vi "self-balance_interface.vi"() -> ()   [LabVIEW 2019]
uses:
  65a3cf9d-86d2-4813-94bd-8b89f2547100.vi
  1c29e484-c04a-4e29-ad32-b5bb79577eec.vi
  <vilib>/Instr/_visa.llb/VISA Configure Serial Port (Instr).vi
  <vilib>/express/express shared/transition.llb/Dynamic To Waveform Array.vi
  <vilib>/express/express signal manip/GetorSetDDTAttributes/Set DDT Attributes/SetT0.vi
  <vilib>/express/express shared/transition.llb/Waveform Array To Dynamic.vi
  <vilib>/express/express signal manip/GetorSetDDTAttributes/Set DDT Attributes/Set DDT Properties.xnode
panel:
  in  "baud rate (9600)":u32=115200
  in  "Salva su Excel":bool
  in  "Percorso file":path=path "C:/Users/d.bevilacqua/Desktop/Bil.xlsx"
  in  "contatore_loop":i32=100
  in  "Tab Control":T1(tab)
  out "Accellerometro":dbl(knob) scale=-90.0..90.0
  out "Filtro complementare:":dbl caption="gradi"
  out "Accellerometro:":dbl caption="gradi"
  out "Correzione baricentro:":sgl caption="gradi" format="%#.1f"
  out "Baricentro":dbl(knob) scale=-15.0..15.0
  out "Controllo:":bool
  out "Angolo":dbl(knob)=-0.787992585102927 scale=-30.0..30.0
  out "Batteria":dbl(slide) scale=11.2..12.6
  out "Velocità motori":dbl(knob) scale=-100.0..100.0
  out "Velocità angolare:":dbl(slide) scale=-300.0..300.0
  out "Motori:":dbl caption="%"
  out "Batteria:":dbl caption="Volts" format="%#_3g"
  out "Giroscopio:":dbl caption="gradi/s"
  in  "Frequenza campionamento dati":i32=120 caption="ms" min=48 max=2400 step=1
  out "Traccia batteria":ext(graph)
  out "Traccia errore":ext(graph)
  out "Traccia angolo":cluster{dbl, dbl, dbl}(graph)
  out "Traccia varianza":ext(graph)
  out "Traccia media":cluster{ext, ext}(graph)
  out "Media errore:":dbl format="%.1e"
  out "Varianza errore:":dbl format="%#_2e"
  out "Errore istantaneo:":dbl format="%#_2g"
  in  "Indietro":bool
  in  "Stop":bool
  in  "Destra":bool
  in  "Sinistra":bool
  in  "Avanti":bool
  in  "Proporzionale":sgl(slide)=20.0 min=0 max=35 step=0.1 scale=0.0..35.0 scale format="%#_3f"
  in  "Integrativo":sgl(slide)=1.4699999 min=0 max=2 step=0.01 scale=0.0..2.0 scale format="%#_2f"
  in  "Derivativo":dbl(slide)=50.31000000000001 min=0.0 max=70.0 step=0.01 scale=0.0..70.0 scale format="%#_2f"
  in  "Applica":bool
  in  "Accensione motori":bool=TRUE caption="motori"
  in  "Applica 3":bool
  in  "Applica 2":bool
  out "Lettura Seriale":string
  in  "stop":bool
  in  "PORTA SERIALE":refnum<visa-resource-name>
  # "BIL 6.0"
  # "Inclinazione"
  # "Media e Varianza dell'errore"
  # "Configurazione PID"
  # "Pilotaggio manuale"
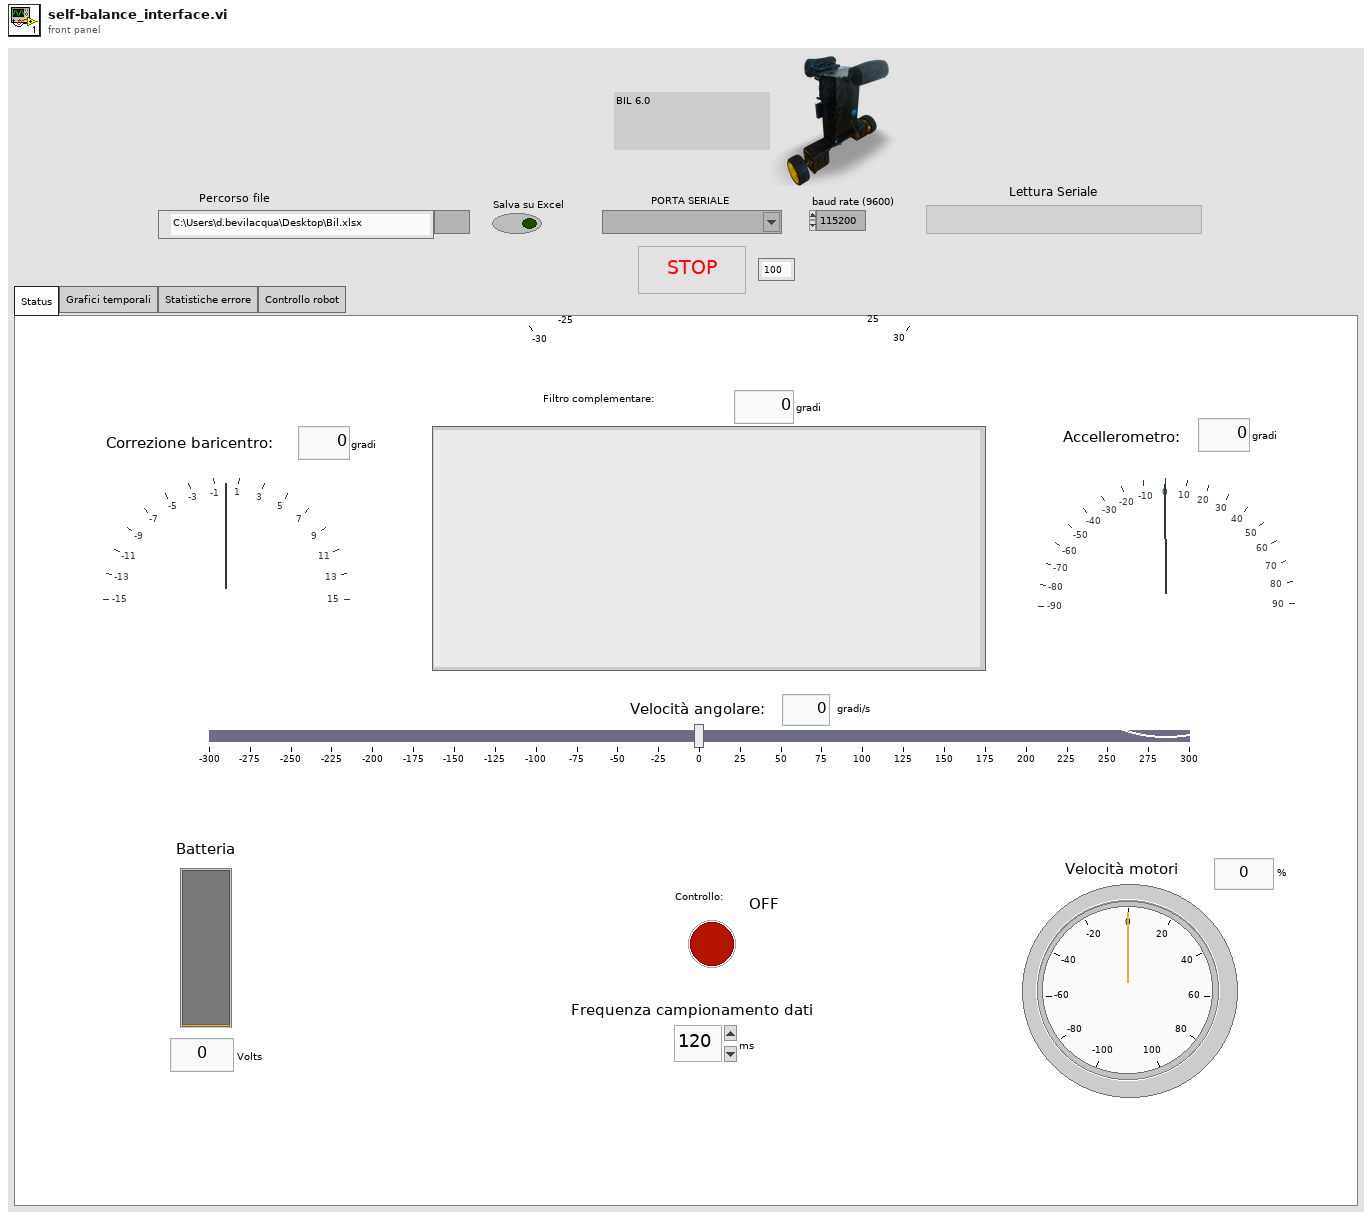
[diagram p1: front panel]
types:
  T1 = enum32{"Status", "Grafici temporali", "Statistiche errore", "Controllo robot"}
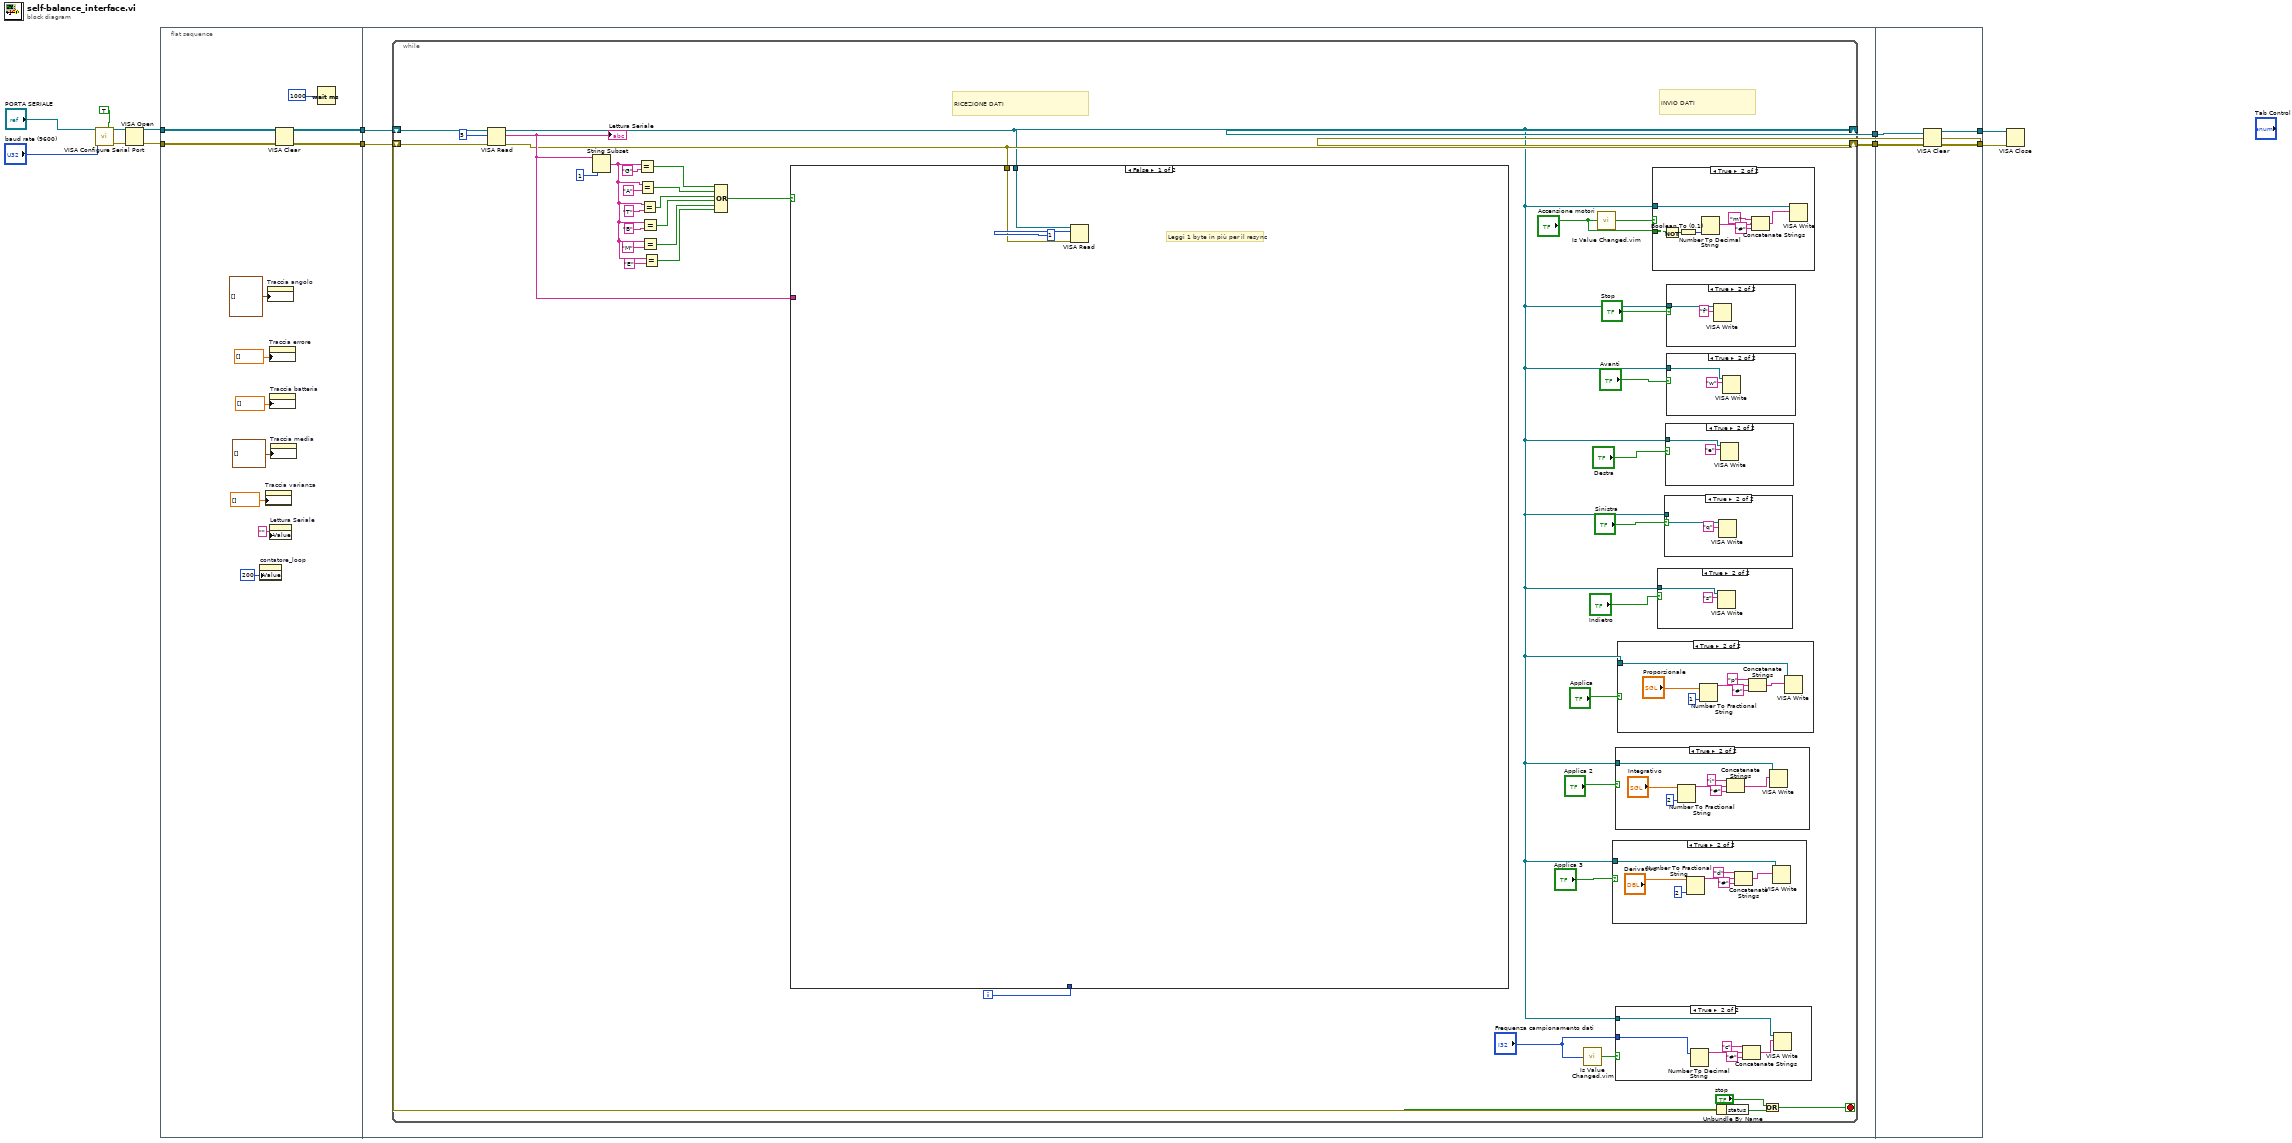
[diagram p0: block diagram]
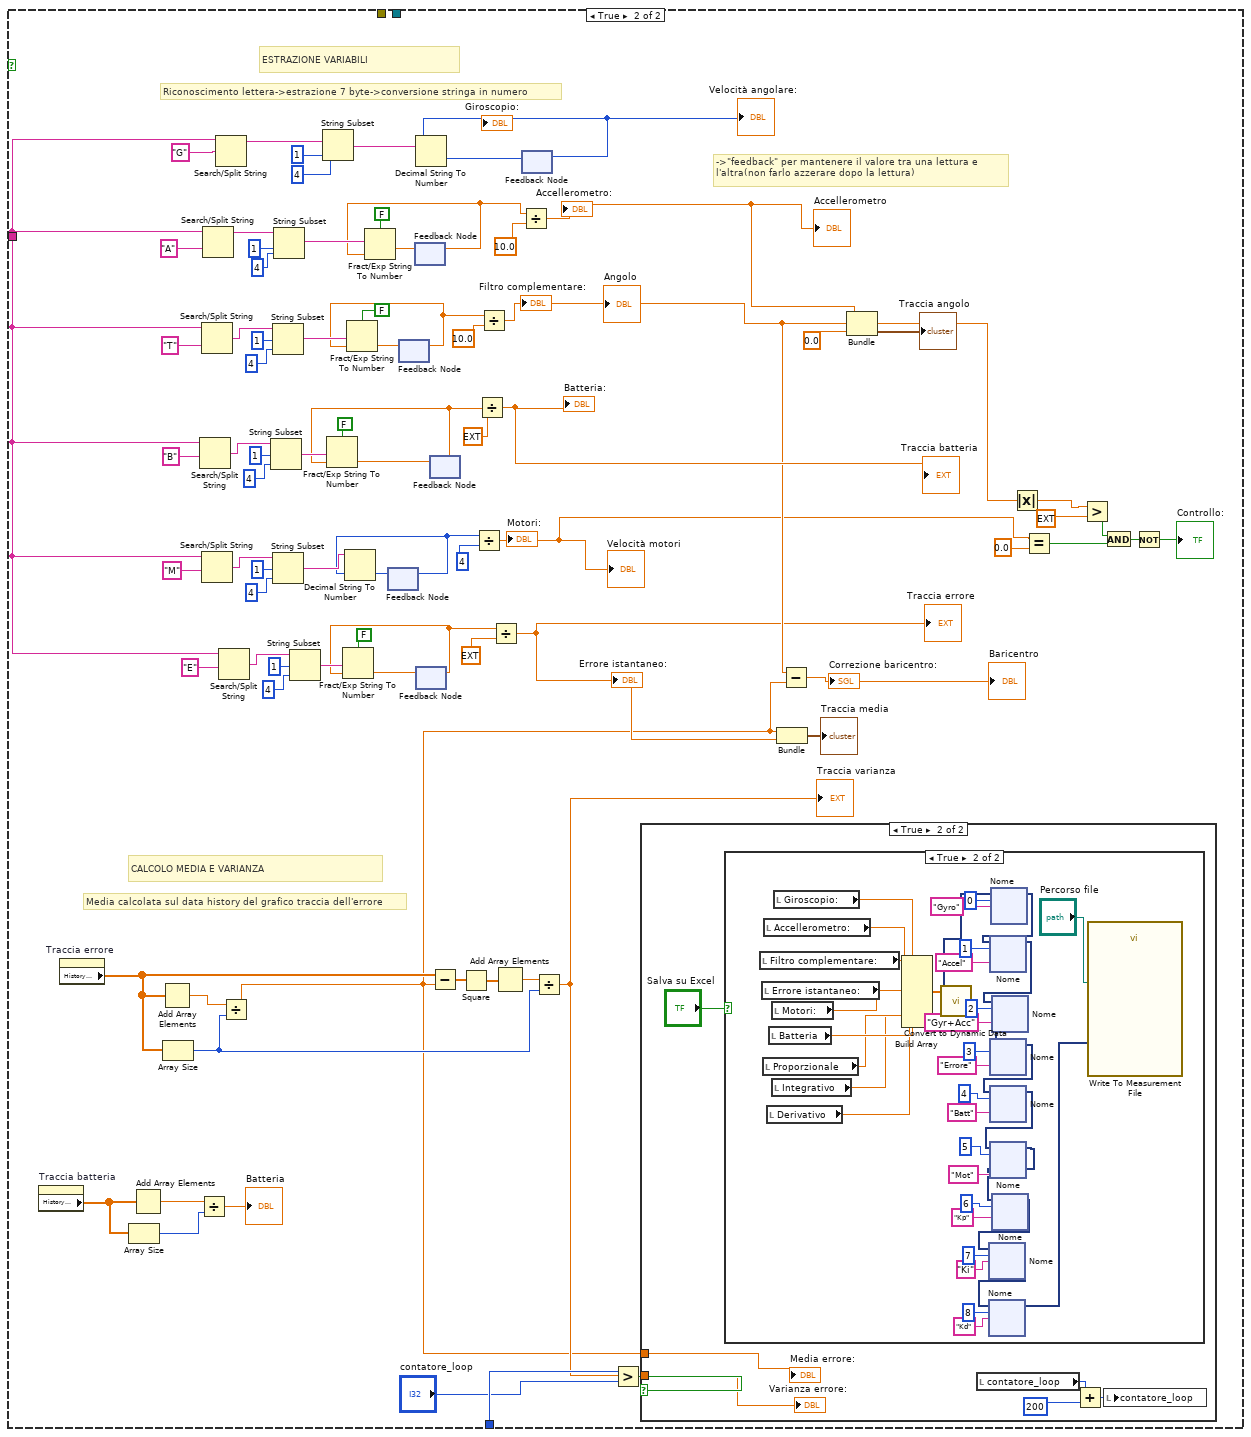
[diagram p10: hidden frame]
diagram:
  n1 = call-poly "VISA Configure Serial Port"("VISA resource name"="PORTA SERIALE", "Enable Termination\nChar (T)"=TRUE, "baud rate (9600)"="baud rate (9600)") -> ("VISA resource name out"=w12:refnum<visa-resource-name>, "error out"=w11:errorcluster)  [unwired: 11 in]
  n2 = VISA Open(error in (no error)=w11, VISA resource name=w12) -> (VISA resource name=w9:refnum<visa-resource-name>, error out=w8:errorcluster)  [unwired: 3 in]
  n3 = flat-sequence {
    tunnel: [w16] -> w3
    tunnel: w9 -> [w24]
    tunnel: w8 -> [w23]
    tunnel: [w15] -> w2
    tunnel: [w27] -> w5
    tunnel: [w26] -> w4
    tunnel: w3 -> [w29]
    tunnel: w2 -> [w28]
    tunnel: [w360] -> w6
    tunnel: [w363] -> w7
    tunnel: w5 -> [w362]
    tunnel: w4 -> [w361]
    frame #0 {
      n4 = property on="contatore_loop" class="DigNum (strict)"("Value"=200 ("contatore_loop")) -> ()  [unwired: 2 in, 2 out]
      n5 = property on="Traccia varianza" class="WFChart (strict)"("History Data"=ext[] []) -> ()  [unwired: 2 in, 2 out]
      n6 = property on="Traccia angolo" class="WFChart (strict)"("History Data"=cluster{ext, ext, dbl}[] []) -> ()  [unwired: 2 in, 2 out]
      n7 = property on="Traccia errore" class="WFChart (strict)"("History Data"=ext[] []) -> ()  [unwired: 2 in, 2 out]
      n8 = property on="Traccia batteria" class="WFChart (strict)"("History Data"=ext[] []) -> ()  [unwired: 2 in, 2 out]
      n9 = property on="Lettura Seriale" class="Str"("Value"="" ("Lettura Seriale")) -> ()  [unwired: 2 in, 2 out]
      n10 = property on="Traccia media" class="WFChart (strict)"("History Data"=cluster{ext, ext}[] []) -> ()  [unwired: 2 in, 2 out]
      n11 = VISA Clear(VISA resource name=w24, error in (no error)=w23) -> (VISA resource name out=w16:refnum<visa-resource-name>, error out=w15:errorcluster)
      n12 = Wait (ms)(milliseconds to wait=u32 1000) -> ()  [unwired: 1 out]
    }
    frame #1 {
      n13 = while {
        shift-right: [w30] -> w27
        shift-left: w29 -> [w65]
        shift-right: [w45] -> w26
        shift-left: w28 -> [w64]
        i -> [w44]
        stop <- w41 stop-if-true
        # "RICEZIONE DATI"
        # "INVIO DATI"
        n14 = VISA Read(VISA resource name=w65, byte count=u32 5, error in (no error)=w64) -> (VISA resource name out=w30:refnum<visa-resource-name>, read buffer=w60:string, error out=w45:errorcluster)  [unwired: 1 out]
        "Lettura Seriale" <- w60
        n15 = String Subset(string=w60, length (rest)=1 ("length (rest)")) -> (substring=w52:string)  [unwired: 1 in]
        n16 = Equal?(x=w52, y="G") -> (x = y?=w58:bool)
        n17 = Equal?(x=w52, y="A") -> (x = y?=w51:bool)
        n18 = Equal?(x=w52, y="T") -> (x = y?=w50:bool)
        n19 = Equal?(x=w52, y="B") -> (x = y?=w49:bool)
        n20 = Equal?(x=w52, y="M") -> (x = y?=w48:bool)
        n21 = Equal?(x=w52, y="E") -> (x = y?=w47:bool)
        n22 = Compound Arithmetic op=OR(w58, w51, w50, w49, w48, w47) -> (w46:bool)
        n23 = case shown="False" w46 {
          tunnel: w60 -> [_ w136]
          tunnel: w30 -> [w98 _]
          tunnel: w45 -> [w97 _]
          tunnel: w44 -> [_ w112]
          frame False {
            # "Leggi 1 byte in più per il resync"
            n24 = VISA Read(VISA resource name=w98, byte count=u32 1, error in (no error)=w97) -> ()  [unwired: 4 out]
          }
          frame True {
            # "->\"feedback\" per mantenere il valore tra una lettura e l'altra(non farlo azzerare dopo la lettura)"
            # "Media calcolata sul data history del grafico traccia dell'errore"
            # "CALCOLO MEDIA E VARIANZA"
            # "Riconoscimento lettera->estrazione 7 byte->conversione stringa in numero"
            # "ESTRAZIONE VARIABILI"
            n25 = property on="Traccia batteria" class="WFChart (strict)"() -> ("History Data"=w118:ext[])  [unwired: 2 in, 2 out]
            n26 = property on="Traccia errore" class="WFChart (strict)"() -> ("History Data"=w113:ext[])  [unwired: 2 in, 2 out]
            n27 = Array Size(array=w118) -> (size(s)=w119:i32)
            n28 = Add Array Elements(numeric array=w118) -> (sum=w120:ext)
            n29 = Add Array Elements(numeric array=w113) -> (sum=w168:ext)
            n30 = Array Size(array=w113) -> (size(s)=w166:i32)
            n31 = Divide(x=w120, y=w119) -> (x/y=→"Batteria":ext)
            n32 = Search/Split String(string=w136, search string/char (-)="B") -> (match + rest of string=w173:string)  [unwired: 1 in, 2 out]
            n33 = Search/Split String(string=w136, search string/char (-)="T") -> (match + rest of string=w177:string)  [unwired: 1 in, 2 out]
            n34 = Search/Split String(string=w136, search string/char (-)="M") -> (match + rest of string=w162:string)  [unwired: 1 in, 2 out]
            n35 = Search/Split String(string=w136, search string/char (-)="A") -> (match + rest of string=w181:string)  [unwired: 1 in, 2 out]
            n36 = Search/Split String(string=w136, search string/char (-)="G") -> (match + rest of string=w155:string)  [unwired: 1 in, 2 out]
            n37 = Search/Split String(string=w136, search string/char (-)="E") -> (match + rest of string=w141:string)  [unwired: 1 in, 2 out]
            n38 = Divide(x=w168, y=w166) -> (x/y=w108:ext)
            n39 = String Subset(string=w173, offset (0)=1, length (rest)=4 ("length (rest)")) -> (substring=w148:string)
            n40 = String Subset(string=w177, offset (0)=1, length (rest)=4 ("length (rest)")) -> (substring=w149:string)
            n41 = String Subset(string=w162, offset (0)=1, length (rest)=4 ("length (rest)")) -> (substring=w159:string)
            n42 = String Subset(string=w181, offset (0)=1, length (rest)=4 ("length (rest)")) -> (substring=w158:string)
            n43 = String Subset(string=w141, offset (0)=1, length (rest)=4 ("length (rest)")) -> (substring=w137:string)
            n44 = String Subset(string=w155, offset (0)=1, length (rest)=4 ("length (rest)")) -> (substring=w156:string)
            n45 = feedback #1() -> (w145:i32)  [unwired: 1 in]
            n46 = Decimal String To Number(string=w159, default (0L)=w145) -> (number=w146:i32)  [unwired: 1 in, 1 out]
            n47 = feedback-in #1(w146) -> ()
            n48 = feedback #2() -> (w129:dbl)  [unwired: 1 in]
            n49 = Fract/Exp String To Number(use system decimal point (T)=FALSE, string=w149, default (0 dbl)=w129) -> (number=w130:dbl)  [unwired: 1 in, 1 out]
            n50 = feedback-in #2(w130) -> ()
            n51 = feedback #3() -> (w131:dbl)  [unwired: 1 in]
            n52 = Fract/Exp String To Number(use system decimal point (T)=FALSE, string=w158, default (0 dbl)=w131) -> (number=w132:dbl)  [unwired: 1 in, 1 out]
            n53 = feedback-in #3(w132) -> ()
            n54 = feedback #4() -> (w128:ext)  [unwired: 1 in]
            n55 = Fract/Exp String To Number(use system decimal point (T)=FALSE, string=w137, default (0 dbl)=w128) -> (number=w123:ext)  [unwired: 1 in, 1 out]
            n56 = feedback-in #4(w123) -> ()
            n57 = feedback #5() -> (w125:ext)  [unwired: 1 in]
            n58 = Fract/Exp String To Number(use system decimal point (T)=FALSE, string=w148, default (0 dbl)=w125) -> (number=w122:ext)  [unwired: 1 in, 1 out]
            n59 = feedback-in #5(w122) -> ()
            n60 = Subtract(x=w113, y=w108) -> (x-y=w167:ext[])
            n61 = Square(x=w167) -> (x^2=w165:ext[])
            n62 = Divide(x=w145, y=4) -> (x/y=w106:dbl)
            "Motori:" <- w106
            "Velocità motori" <- w106
            n63 = Divide(x=w125, y=ext 10.0) -> (x/y=→"Batteria:" →"Traccia batteria":ext)
            n64 = Divide(x=w129, y=10.0) -> (x/y=w116:dbl)
            "Angolo" <- w116
            "Filtro complementare:" <- w116
            n65 = Divide(x=w128, y=ext 10.0) -> (x/y=w114:ext)
            "Traccia errore" <- w114
            "Errore istantaneo:" <- w114
            n66 = Add Array Elements(numeric array=w165) -> (sum=w164:ext)
            n67 = Divide(x=w131, y=10.0) -> (x/y=w117:dbl)
            "Accellerometro" <- w117
            "Accellerometro:" <- w117
            n68 = feedback #6() -> (w143:i32)  [unwired: 1 in]
            "Giroscopio:" <- w143
            "Velocità angolare:" <- w143
            n69 = Decimal String To Number(string=w156, default (0L)=w143) -> (number=w144:i32)  [unwired: 1 in, 1 out]
            n70 = feedback-in #6(w144) -> ()
            n71 = Divide(x=w164, y=w166) -> (x/y=w109:ext)
            "Traccia varianza" <- w109
            n72 = Greater?(x=w112, y="contatore_loop") -> (0:w110:bool)
            n73 = case shown="True" w110 {
              tunnel: w108 -> [_ w185]
              tunnel: w109 -> [_ w184]
              frame False {
              }
              frame True {
                n74 = case shown="True" "Salva su Excel" {
                  frame False {
                  }
                  frame True {
                    n75 = local read "Filtro complementare:"() -> (w225:dbl)
                    n76 = local read "Errore istantaneo:"() -> (w224:dbl)
                    n77 = local read "Proporzionale"() -> (w221:sgl)
                    n78 = local read "Accellerometro:"() -> (w226:dbl)
                    n79 = local read "Derivativo"() -> (w219:dbl)
                    n80 = local read "Batteria"() -> (w222:dbl)
                    n81 = local read "Motori:"() -> (w223:dbl)
                    n82 = local read "Integrativo"() -> (w220:sgl)
                    n83 = local read "Giroscopio:"() -> (w227:dbl)
                    n84 = Build Array(w227, w226, w225, w224, w223, w222, w221, w220, w219) -> (w218:dbl[])
                    n85 = call "Convert to Dynamic Data"("Array"=w218) -> ("Dynamic Data Type"=w217:dynamicdata)  [unwired: 3 in]
                    n86 = xnode "Nome"("Signals In"=w217, "Signal Index"=0, "Signal Name"="Gyro") -> ("Signals Out"=w206:dynamicdata)  [unwired: 1 in, 1 out]
                    n87 = xnode "Nome"("Signals In"=w206, "Signal Index"=1, "Signal Name"="Accel") -> ("Signals Out"=w205:dynamicdata)  [unwired: 1 in, 1 out]
                    n88 = xnode "Nome"("Signals In"=w205, "Signal Index"=2, "Signal Name"="Gyr+Acc") -> ("Signals Out"=w204:dynamicdata)  [unwired: 1 in, 1 out]
                    n89 = xnode "Nome"("Signals In"=w204, "Signal Index"=3, "Signal Name"="Errore") -> ("Signals Out"=w203:dynamicdata)  [unwired: 1 in, 1 out]
                    n90 = xnode "Nome"("Signals In"=w203, "Signal Index"=4, "Signal Name"="Batt") -> ("Signals Out"=w199:dynamicdata)  [unwired: 1 in, 1 out]
                    n91 = xnode "Nome"("Signals In"=w199, "Signal Index"=5, "Signal Name"="Mot") -> ("Signals Out"=w197:dynamicdata)  [unwired: 1 in, 1 out]
                    n92 = xnode "Nome"("Signals In"=w197, "Signal Index"=6, "Signal Name"="Kp") -> ("Signals Out"=w194:dynamicdata)  [unwired: 1 in, 1 out]
                    n93 = xnode "Nome"("Signals In"=w194, "Signal Index"=7, "Signal Name"="Ki") -> ("Signals Out"=w193:dynamicdata)  [unwired: 1 in, 1 out]
                    n94 = xnode "Nome"("Signals In"=w193, "Signal Index"=8, "Signal Name"="Kd") -> ("Signals Out"=w192:dynamicdata)  [unwired: 1 in, 1 out]
                    n95 = call "Write To Measurement File"("Signals"=w192, "Filename"="Percorso file") -> ()  [unwired: 15 in, 3 out]
                  }
                }
                n96 = local read "contatore_loop"() -> (w187:i32)
                n97 = Add(x=w187, y=200) -> (x+y=w188:i32)
                n98 = local write "contatore_loop"(w188) -> ()
                "Media errore:" <- w185
                "Varianza errore:" <- w184
              }
            }
            n99 = Bundle(w108, w114) -> (→"Traccia media":cluster{ext, ext})  [unwired: 1 in]
            n100 = Subtract(x=w116, y=w108) -> (x-y=→"Baricentro" →"Correzione baricentro:":ext)
            n101 = Bundle(w117, w116, 0.0) -> (→"Traccia angolo":cluster{dbl, dbl, dbl})  [unwired: 1 in]
            n102 = Absolute Value(x=w116) -> (abs(x)=w104:dbl)
            n103 = Equal?(x=w106, y=0.0) -> (x = y?=w107:bool)
            n104 = Greater?(x=w104, y=ext 35.0) -> (0:w102:bool)
            n105 = And(x=w102, y=w107) -> (x .and. y?=w101:bool)
            n106 = Not(x=w101) -> (.not. x?=→"Controllo:":bool)
          }
        }
        n107 = call "Is Value Changed.vim"("value"="Frequenza campionamento dati") -> ("changed or first call?"=w32:bool)
        n108 = call "Is Value Changed.vim"("value"="Accensione motori") -> ("changed or first call?"=w63:bool)
        n109 = case shown="True" "Applica 3" {
          tunnel: w30 -> [_ w74]
          frame False {
          }
          frame True {
            n110 = Number To Fractional String(number="Derivativo", precision (6)=i16 2) -> (F-format string=w78:string)  [unwired: 2 in]
            n111 = Concatenate Strings("d" ("write buffer"), w78, "#" ("string")) -> (w73:string)
            n112 = VISA Write(VISA resource name=w74, write buffer=w73) -> ()  [unwired: 1 in, 3 out]
          }
        }
        n113 = case shown="True" "Applica 2" {
          tunnel: w30 -> [_ w81]
          frame False {
          }
          frame True {
            n114 = Number To Fractional String(number="Integrativo", precision (6)=i16 2) -> (F-format string=w85:string)  [unwired: 2 in]
            n115 = Concatenate Strings("i" ("write buffer"), w85, "#" ("string")) -> (w80:string)
            n116 = VISA Write(VISA resource name=w81, write buffer=w80) -> ()  [unwired: 1 in, 3 out]
          }
        }
        n117 = case shown="True" w32 {
          tunnel: "Frequenza campionamento dati" -> [_ w69]
          tunnel: w30 -> [_ w67]
          frame False {
          }
          frame True {
            n118 = Number To Decimal String(number=w69) -> (decimal integer string=w72:string)  [unwired: 1 in]
            n119 = Concatenate Strings("c" ("write buffer"), w72, "#" ("string")) -> (w68:string)
            n120 = VISA Write(VISA resource name=w67, write buffer=w68) -> ()  [unwired: 1 in, 3 out]
          }
        }
        n121 = case shown="True" "Applica" {
          tunnel: w30 -> [_ w355]
          frame False {
          }
          frame True {
            n122 = Number To Fractional String(number="Proporzionale", precision (6)=i16 1) -> (F-format string=w358:string)  [unwired: 2 in]
            n123 = Concatenate Strings("p" ("write buffer"), w358, "#" ("string")) -> (w353:string)
            n124 = VISA Write(VISA resource name=w355, write buffer=w353) -> ()  [unwired: 1 in, 3 out]
          }
        }
        n125 = case shown="True" w63 {
          tunnel: w30 -> [_ w352]
          tunnel: "Accensione motori" -> [_ w345]
          frame False {
          }
          frame True {
            n126 = Not(x=w345) -> (.not. x?=w346:bool)
            n127 = Boolean To (0,1)(Boolean=w346) -> (0, 1=w349:i16)
            n128 = Number To Decimal String(number=w349) -> (decimal integer string=w348:string)  [unwired: 1 in]
            n129 = Concatenate Strings("m" ("write buffer"), w348, "#" ("string")) -> (w351:string)
            n130 = VISA Write(VISA resource name=w352, write buffer=w351) -> ()  [unwired: 1 in, 3 out]
          }
        }
        n131 = case shown="True" "Indietro" {
          tunnel: w30 -> [_ w87]
          frame False {
          }
          frame True {
            n132 = VISA Write(VISA resource name=w87, write buffer="s") -> ()  [unwired: 1 in, 3 out]
          }
        }
        n133 = case shown="True" "Sinistra" {
          tunnel: w30 -> [_ w89]
          frame False {
          }
          frame True {
            n134 = VISA Write(VISA resource name=w89, write buffer="q") -> ()  [unwired: 1 in, 3 out]
          }
        }
        n135 = case shown="True" "Destra" {
          tunnel: w30 -> [_ w91]
          frame False {
          }
          frame True {
            n136 = VISA Write(VISA resource name=w91, write buffer="e") -> ()  [unwired: 1 in, 3 out]
          }
        }
        n137 = case shown="True" "Avanti" {
          tunnel: w30 -> [_ w93]
          frame False {
          }
          frame True {
            n138 = VISA Write(VISA resource name=w93, write buffer="w") -> ()  [unwired: 1 in, 3 out]
          }
        }
        n139 = case shown="True" "Stop" {
          tunnel: w30 -> [_ w96]
          frame False {
          }
          frame True {
            n140 = VISA Write(VISA resource name=w96, write buffer="f") -> ()  [unwired: 1 in, 3 out]
          }
        }
        n141 = Unbundle By Name(w64) -> ("status"=w43:bool)
        n142 = Or(x="stop", y=w43) -> (x .or. y?=w41:bool)
      }
    }
    frame #2 {
      n143 = VISA Clear(VISA resource name=w362, error in (no error)=w361) -> (VISA resource name out=w363:refnum<visa-resource-name>, error out=w360:errorcluster)
    }
  }
  n144 = VISA Close(VISA resource name=w7, error in (no error)=w6) -> ()  [unwired: 1 out]
